vi "set_config_cluster.vi"(8 "error in (no error)":errorcluster, 10 "config cluster variant":variant, 11 "StageDL090602SutterMP285 in":refnum<class "StageMMS2015ASI.lvclass">) -> (0 "error out":errorcluster, 3 "StageDL090602SutterMP285 out":refnum<class "StageMMS2015ASI.lvclass">)   [LabVIEW 2010, in "StageMMS2015ASI.lvclass"]
uses:
  StageMMS2015ASI.lvclass
  StageMMS2015ASI.lvclass/StageMMS2015ASI.ctl
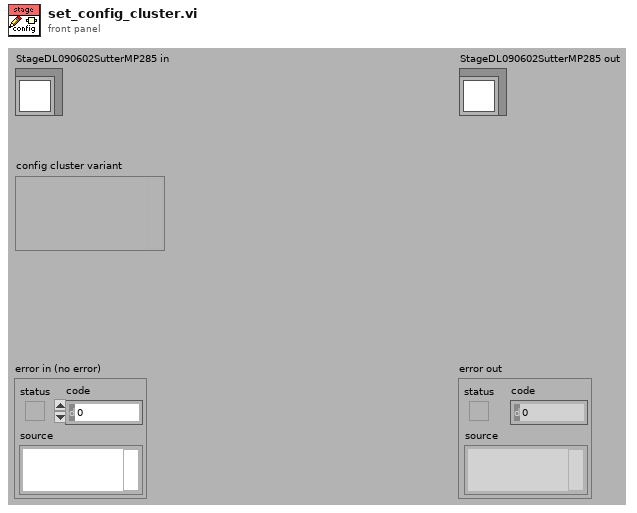
[diagram p1: front panel]
types:
  T1 = typedef "StageMMS2015ASI.lvclass/config_data_cluster.ctl" = cluster{"serial port":string, "speed":dbl[unit], "step factor":dbl[unit]}
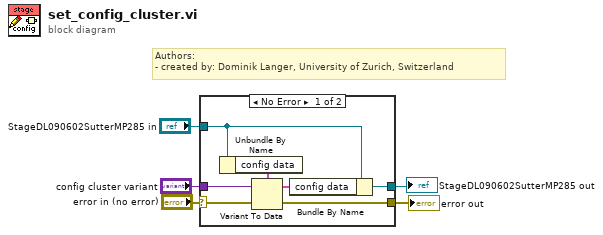
[diagram p0: block diagram]
diagram:
  # "Authors: \n- created by: Dominik Langer, University of Zurich, Switzerland"
  n1 = case shown="No Error" "error in (no error)" {
    selector: "error in (no error)" -> [w10 w13]
    tunnel: "StageDL090602SutterMP285 in" -> [w6 w14]
    tunnel: [w8 w13] -> w1
    tunnel: [w7 w14] -> w2
    tunnel: "config cluster variant" -> [w9 _]
    frame No Error {
      n2 = Unbundle By Name(w6) -> ("config data"=w12:T1)
      n3 = Variant To Data(error in=w10, Variant=w9, type=w12) -> (error out=w8:errorcluster, data=w11:T1)
      n4 = Bundle By Name(cluster=w6, "config data"=w11) -> (w7:refnum<class "StageMMS2015ASI.lvclass">)
    }
    frame Error {
    }
  }
  "error out" <- w1
  "StageDL090602SutterMP285 out" <- w2
